vi "Resample.vi"(8 "error in (no error)":errorcluster, 11 "DSP in":refnum<class "DSP.lvclass">) -> (0 "error out":errorcluster, 2 "Waveforms":T1, 3 "DSP out":refnum<class "DSP.lvclass">, 5 "Continue DSP?":bool)   [LabVIEW 2019, in "DSP.lvclass"]
uses:
  DSP.lvclass
panel:
  out "Waveforms in":T1
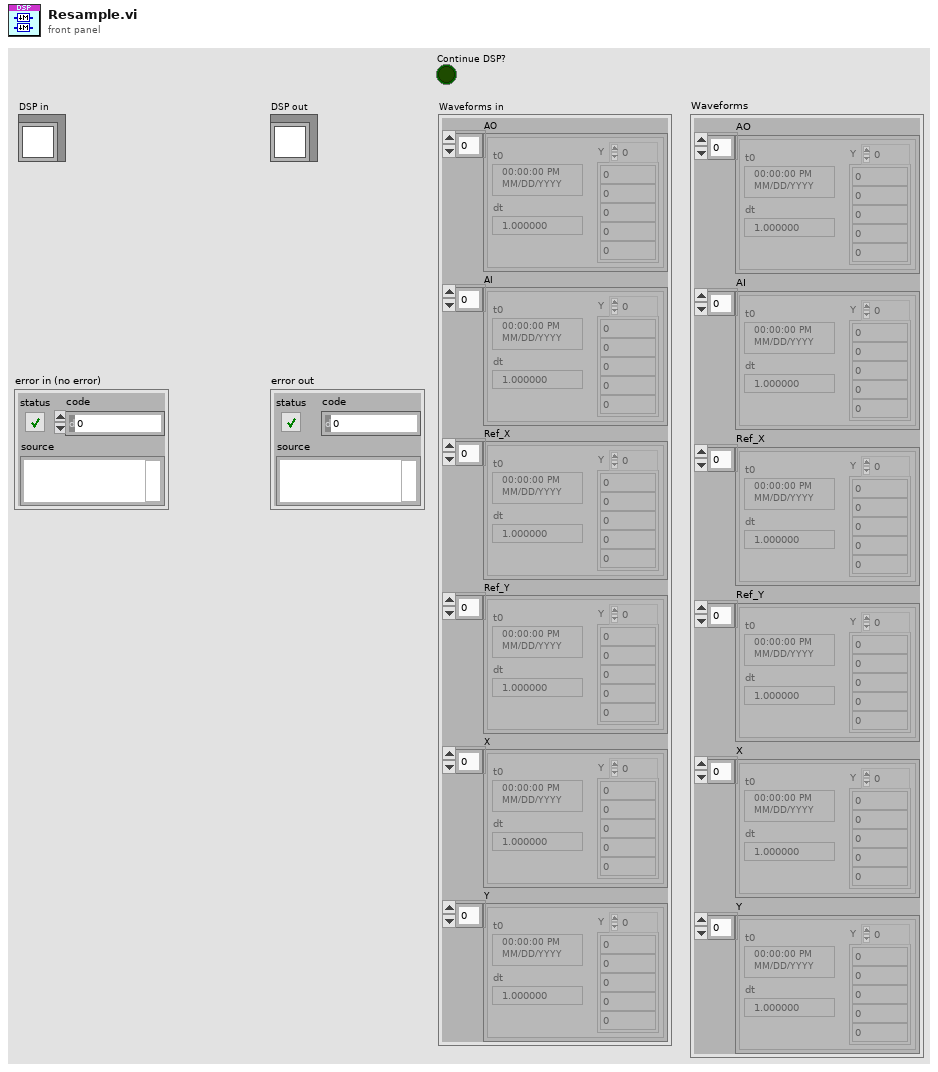
[diagram p1: front panel]
types:
  T1 = cluster{"AO":waveform(dbl)[], "AI":waveform(dbl)[], "Ref_X":waveform(dbl)[], "Ref_Y":waveform(dbl)[], "X":waveform(dbl)[], "Y":waveform(dbl)[]}
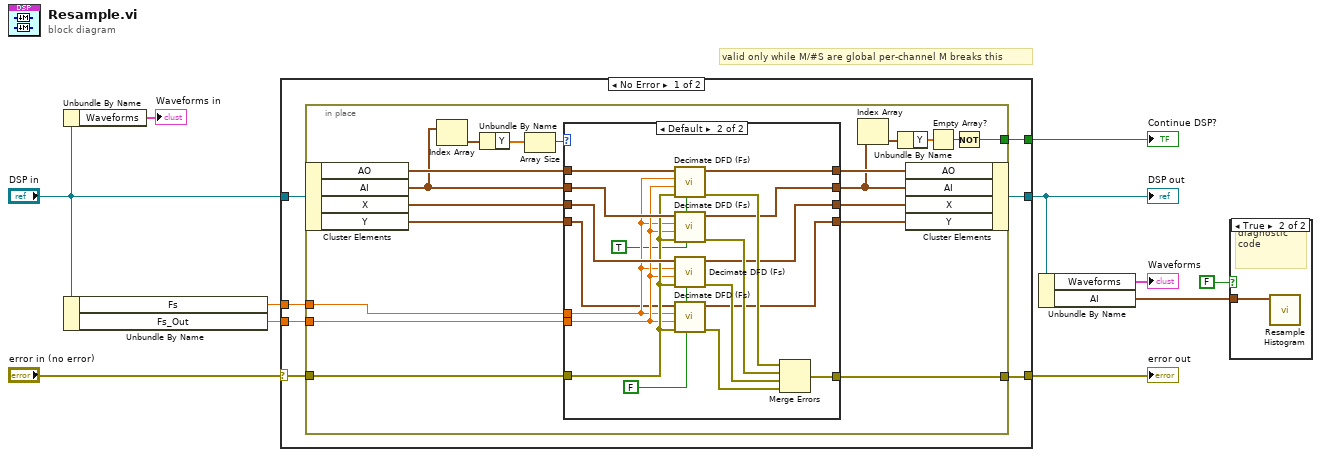
[diagram p0: block diagram]
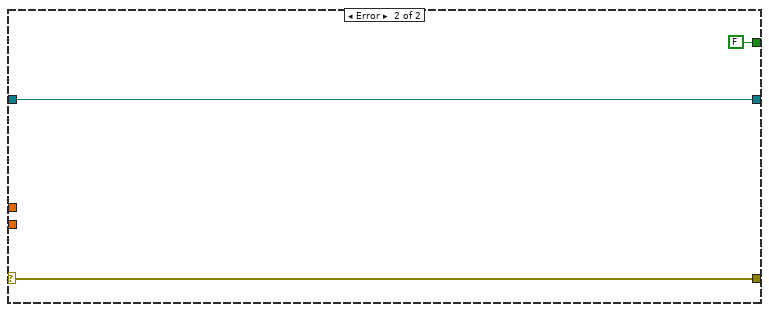
[diagram p3: hidden frame]
diagram:
  # "valid only while M/#S are global per-channel M breaks this"
  n1 = Unbundle By Name("DSP in") -> ("Waveforms"=→"Waveforms in":T1)
  n2 = Unbundle By Name("DSP in") -> ("Fs"=w8:dbl, "Fs_Out"=w9:dbl)
  n3 = case shown="No Error" "error in (no error)" {
    selector: "error in (no error)" -> [w18 w63]
    tunnel: [w16 w63] -> w10
    tunnel: "DSP in" -> [w17 w62]
    tunnel: [w15 w62] -> w7
    tunnel: w9 -> [w14 _]
    tunnel: w8 -> [w13 _]
    tunnel: [w12 FALSE] -> w1
    frame No Error {
      n4 = in-place {
        in-place-border: w18 -> [w33]
        in-place-border: [w37] -> w16
        in-place-border: w14 -> [w32]
        in-place-border: w13 -> [w31]
        in-place-border: [w19] -> w12
        n5 = in-place-cluster #1(w17) -> ("AO"=w36:waveform(dbl)[], "AI"=w25:waveform(dbl)[], "X"=w35:waveform(dbl)[], "Y"=w29:waveform(dbl)[])
        n6 = Index Array(array=w25) -> (element=w28:waveform(dbl))  [unwired: 1 in]
        n7 = Unbundle By Name(w28) -> ("Y"=w27:dbl[])
        n8 = Array Size(array=w27) -> (size(s)=w26:i32)
        n9 = case shown="Default" w26 {
          tunnel: [w38 w60] -> w37
          tunnel: w36 -> [w42 w55]
          tunnel: w25 -> [w41 w54]
          tunnel: w35 -> [w39 w53]
          tunnel: [w42 w52] -> w24
          tunnel: [w40 w51] -> w34
          tunnel: w33 -> [w38 w50]
          tunnel: w32 -> [_ w49]
          tunnel: w31 -> [_ w48]
          tunnel: [w41 w47] -> w22
          tunnel: [w39 w46] -> w30
          tunnel: w29 -> [w40 w45]
          frame 0, 1 {
          }
          frame Default {
            w43 = FALSE ("Nyquist Filter [F]")
            w44 = TRUE ("Nyquist Filter [F]")
            n10 = call "Decimate DFD (Fs).vi"("Nyquist Filter [F]"=w44, "error in (no error)"=w50, "output fs (Hz)"=w49, "Fs"=w48, "Waveforms in"=w55) -> ("error out"=w59:errorcluster, "waveforms out"=w52:waveform(dbl)[])  [unwired: 5 in]
            n11 = call "Decimate DFD (Fs).vi"("Nyquist Filter [F]"=w44, "error in (no error)"=w50, "output fs (Hz)"=w49, "Fs"=w48, "Waveforms in"=w54) -> ("error out"=w58:errorcluster, "waveforms out"=w47:waveform(dbl)[])  [unwired: 5 in]
            n12 = call "Decimate DFD (Fs).vi"("Nyquist Filter [F]"=w43, "error in (no error)"=w50, "output fs (Hz)"=w49, "Fs"=w48, "Waveforms in"=w53) -> ("error out"=w57:errorcluster, "waveforms out"=w46:waveform(dbl)[])  [unwired: 5 in]
            n13 = call "Decimate DFD (Fs).vi"("Nyquist Filter [F]"=w43, "error in (no error)"=w50, "output fs (Hz)"=w49, "Fs"=w48, "Waveforms in"=w45) -> ("error out"=w56:errorcluster, "waveforms out"=w51:waveform(dbl)[])  [unwired: 5 in]
            n14 = Merge Errors(w59, w58, w57, w56) -> (w60:errorcluster)
          }
        }
        n15 = Index Array(array=w22) -> (element=w23:waveform(dbl))  [unwired: 1 in]
        n16 = Unbundle By Name(w23) -> ("Y"=w21:dbl[])
        n17 = in-place-cluster #1("AO"=w24, "AI"=w22, "X"=w30, "Y"=w34) -> (w15:refnum<class "DSP.lvclass">)
        n18 = Empty Array?(array=w21) -> (empty?=w20:bool)
        n19 = Not(x=w20) -> (.not. x?=w19:bool)
      }
    }
    frame Error {
    }
  }
  "error out" <- w10
  "DSP out" <- w7
  "Continue DSP?" <- w1
  n20 = Unbundle By Name(w7) -> ("Waveforms"=→"Waveforms":T1, "AI"=w3:waveform(dbl)[])
  n21 = case shown="True" FALSE {
    tunnel: w3 -> [_ w64]
    frame False {
    }
    frame True {
      # "diagnostic code"
      n22 = call "Resample Histogram.vi"("AI"=w64) -> ()  [unwired: 11 in]
    }
  }
